vi "viewStatus.vi"(8 "error in (no error)":errorcluster, 11 "MissionQueue in":refnum<class "MissionQueue.lvclass">) -> (0 "error out":errorcluster, 1 "Queue length":i32, 2 "Is empty?":bool, 3 "MissionQueue out":refnum<class "MissionQueue.lvclass">)   [LabVIEW 2011, in "MissionQueue.lvclass"]
doc: "Views the mission queue and returns how many elements the queue contains and whether or not it is empty."
uses:
  MissionQueue.lvclass
  MissionQueue.lvclass/MissionQueue.ctl
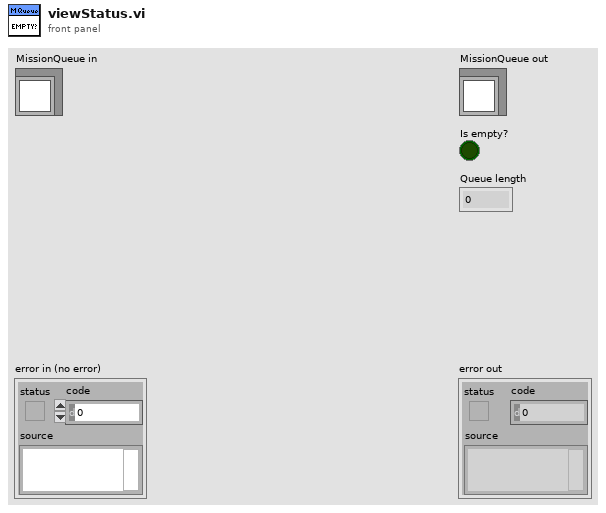
[diagram p1: front panel]
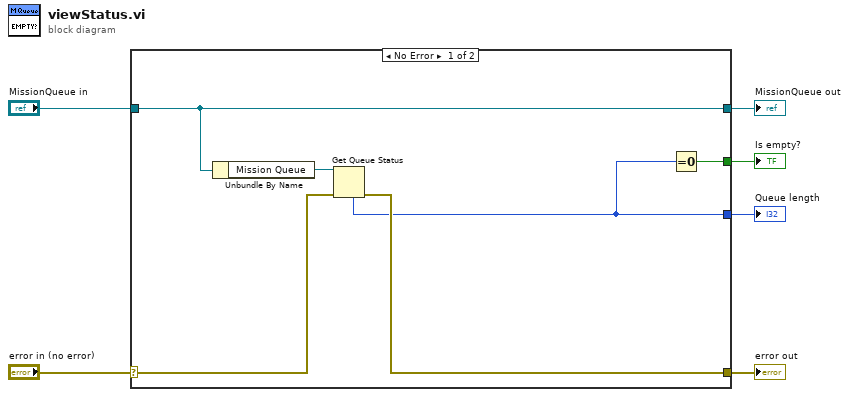
[diagram p0: block diagram]
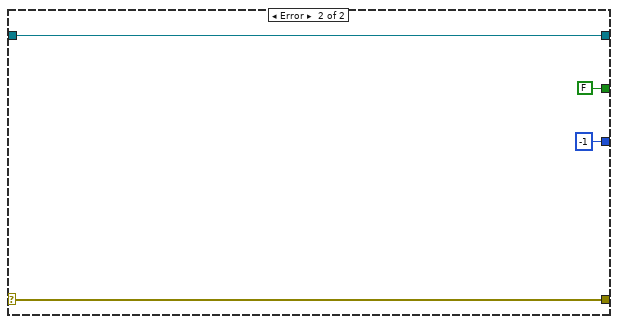
[diagram p2: hidden frame]
diagram:
  n1 = case shown="No Error" "error in (no error)" {
    selector: "error in (no error)" -> [w10 w16]
    tunnel: [w9 w16] -> w5
    tunnel: [w12 w15] -> w3
    tunnel: "MissionQueue in" -> [w12 w15]
    tunnel: [w8 FALSE] -> w2
    tunnel: [w7 -1 ("# elements in queue")] -> w1
    frame No Error {
      n2 = Unbundle By Name(w12) -> ("Mission Queue"=w11:refnum<queue>)
      n3 = Get Queue Status(queue=w11, error in (no error)=w10) -> (error out=w9:errorcluster, # elements in queue=w7:i32)  [unwired: 1 in, 6 out]
      n4 = Equal To 0?(x=w7) -> (x = 0?=w8:bool)
    }
    frame Error {
    }
  }
  "error out" <- w5
  "MissionQueue out" <- w3
  "Is empty?" <- w2
  "Queue length" <- w1
